vi "VITester_Item_OnPopupMenu.vi"(11 "Object":T1) -> ()   [LabVIEW 2009]
uses:
  Support/VITester Project Item Ref.ctl
panel:
  out "error out":errorcluster
  in  "error in":errorcluster
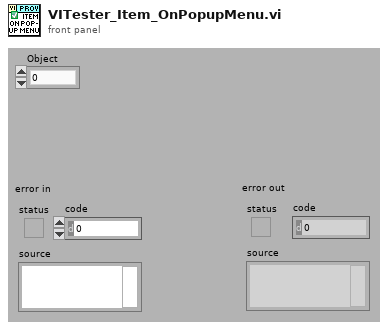
[diagram p1: front panel]
types:
  T1 = typedef "VITester Project Item Ref.ctl" = u64
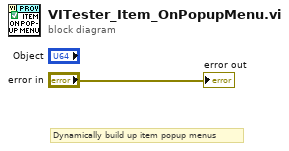
[diagram p0: block diagram]
diagram:
  # "Dynamically build up item popup menus"
  "error out" <- "error in"
